vi "Convert GPS To Table Array.vi"(1 "Waypoint Array In":T1(array[cluster]) {"Time"."GPS Time of Week" format="%.3f"; "Velocity, Correction & SET"."Extended Navigation Mode" items=["Non Differential"=0, "Code (RTCM Type 1 & 9)"=1, "Code, Single Frequency (WAAS)"=2, "Code, Dual Frequency (WAAS)"=3, "Code, Single Frequency (WCT)"=4, "Code/RCP, Dual Frequency (WCT)"=5, "Code, Single Frequency (RTG)"=6, "Code (RTCM Type 1 & 9) Dual Frequency"=10, "Code/RCP, Dual Frequency (RTG)"=11, "Code, Single Frequency (NCT-RTK)"=12, "Code, Single Frequency (RTCM 18 & 19)"=13, "Code, Single Frequency (RTCM 21 & 22)"=14, "Code, Single Frequency (CMR)"=15, "Code, Dual Frequency (NCT-RTK)"=16, "Code, Dual Frequency (RTCM 18 & 19)"=17, "Code, Dual Frequency (RTCM 20 & 21)"=18, "Code, Dual Frequency (CMR)"=19, "RTK (NCT-RTK)"=20, "RTK (RTCM 18 & 19)"=21, "RTK (RTCM 20 & 21)"=22, "RTK (CMR)"=23, "Code, Single Frequency with SET (RTG)"=24, "Code/RCP, Dual Frequency with SET (RTG)"=25, "RTK Extend"=26]}) -> (0 "Lat/Long Array Out":string[][](array[string]))   [LabVIEW 2012]
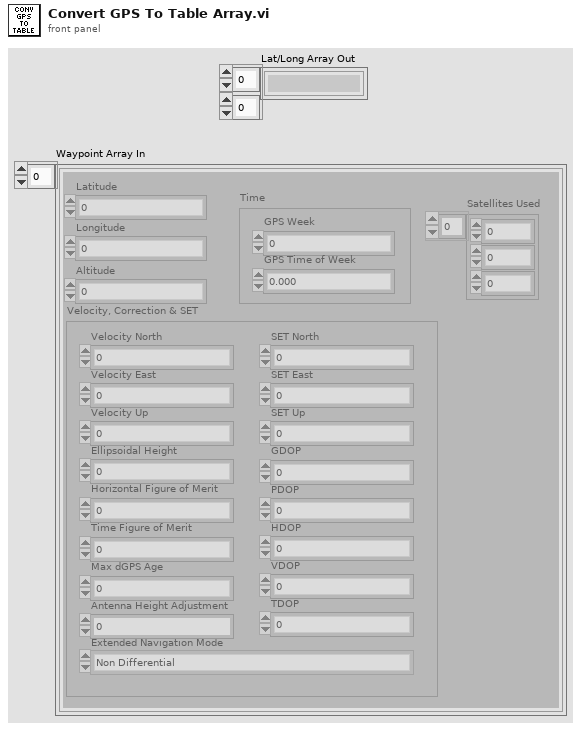
[diagram p1: front panel]
types:
  T1 = cluster{"Latitude":dbl, "Longitude":dbl, "Altitude":dbl, "Velocity, Correction & SET":cluster{"Velocity North":dbl, "Velocity East":dbl, "Velocity Up":dbl, "Ellipsoidal Height":dbl, "GDOP":sgl, "PDOP":sgl, "HDOP":sgl, "VDOP":sgl, "TDOP":sgl, "Horizontal Figure of Merit":u8, "Time Figure of Merit":u8, "Max dGPS Age":sgl, "Extended Navigation Mode":u8, "Antenna Height Adjustment ":dbl, "SET North":i32, "SET East":i32, "SET Up":i32}, "Time":cluster{"GPS Week":u16, "GPS Time of Week":sgl}, "Satellites Used":i32[]}[]
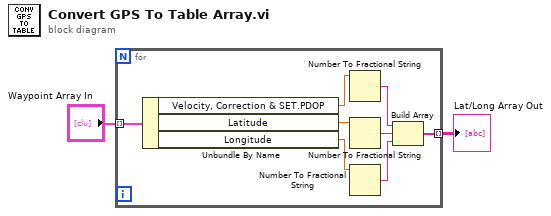
[diagram p0: block diagram]
diagram:
  n1 = for {
    tunnel: "Waypoint Array In" -> [w10] mode=indexing
    tunnel: [w3] -> w1 mode=indexing
    n2 = Unbundle By Name(w10) -> ("Velocity, Correction & SET.PDOP"=w8:sgl, "Latitude"=w7:dbl, "Longitude"=w9:dbl)
    n3 = Number To Fractional String(number=w8) -> (F-format string=w5:string)  [unwired: 3 in]
    n4 = Number To Fractional String(number=w7) -> (F-format string=w6:string)  [unwired: 3 in]
    n5 = Number To Fractional String(number=w9) -> (F-format string=w4:string)  [unwired: 3 in]
    n6 = Build Array(w5, w6, w4) -> (w3:string[])
  }
  "Lat/Long Array Out" <- w1
